vi "Initialise State.vi"(8 "error in (no error)":errorcluster, 11 "OnChange_Boolean in":refnum<class "OnChangeNotifier_EXT.lvclass">) -> (0 "error out":errorcluster, 3 "OnChange_Boolean out":refnum<class "OnChangeNotifier_EXT.lvclass">)   [LabVIEW 2021, in "OnChangeNotifier_EXT.lvclass"]
uses:
  OnChangeNotifier_EXT.lvclass
  <vilib>/TSA/Abstract Data Classes/Abs_Types/Single Float/Static Read.vi
  <vilib>/TSA/Abstract Data Classes/Abs_Types/Single Float/Abs_Single Float.lvclass
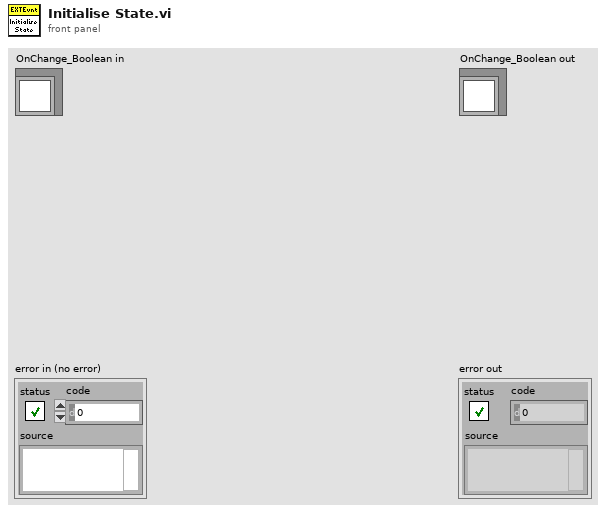
[diagram p1: front panel]
types:
  T1 = typedef "OnChangeNotifier_EXT.lvclass/Class Type.ctl" = refnum<class "Abs_Single Float.lvclass">
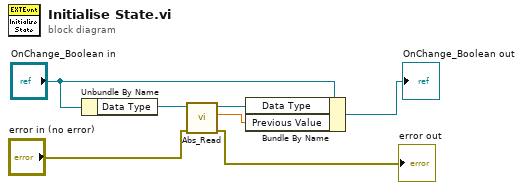
[diagram p0: block diagram]
diagram:
  n1 = Unbundle By Name("OnChange_Boolean in") -> ("Data Type"=w7:T1)
  n2 = call-poly <vilib>:"Abs_Read.vi"("error in (no error)"="error in (no error)", "Abs_Single Float in"=w7) -> ("error out"=→"error out":errorcluster, "Value"=w3:sgl, "Abs_Single Float out"=w5:T1)  [unwired: 7 in]
  n3 = Bundle By Name(cluster="OnChange_Boolean in", "Data Type"=w5, "Previous Value"=w3) -> (→"OnChange_Boolean out":refnum<class "OnChangeNotifier_EXT.lvclass">)
